vi "Arm.vi"(8 "error in (no error)":errorcluster, 11 "Shutter in":refnum<class "Shutter.lvclass">) -> (0 "error out":errorcluster, 2 "State":T1, 3 "Shutter out":refnum<class "Shutter.lvclass">)   [LabVIEW 2016, in "Shutter.lvclass"]
uses:
  Shutter.lvclass
  Controls/Shutter States.ctl
  Shutter.lvclass/Shutter.ctl
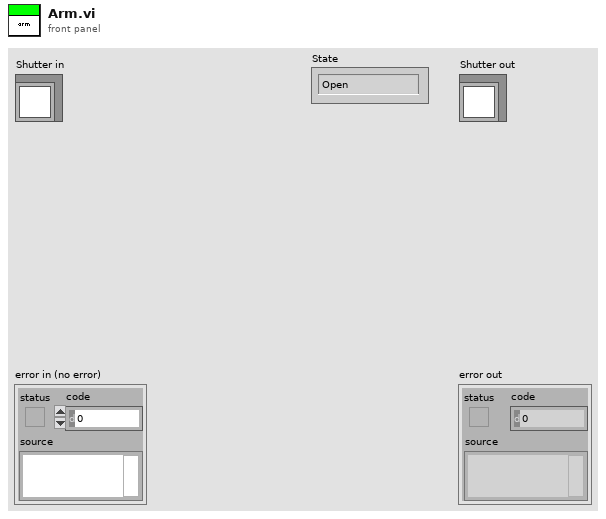
[diagram p1: front panel]
types:
  T1 = typedef "Shutter States.ctl" = enum16{"Open", "Close", "Wait", "Off", "Arm", "Idle"}
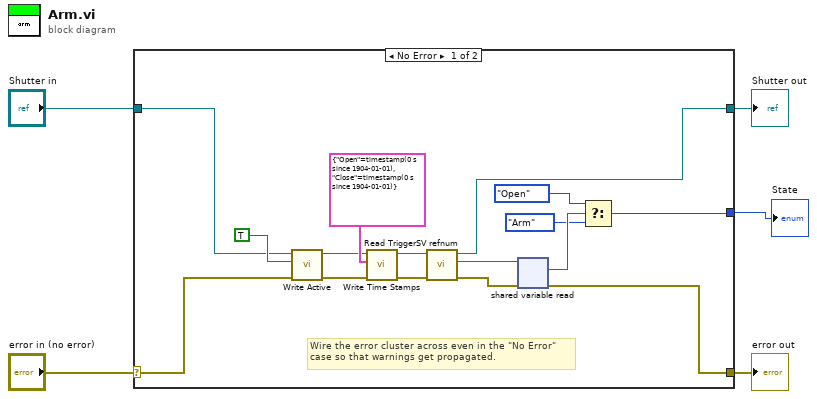
[diagram p0: block diagram]
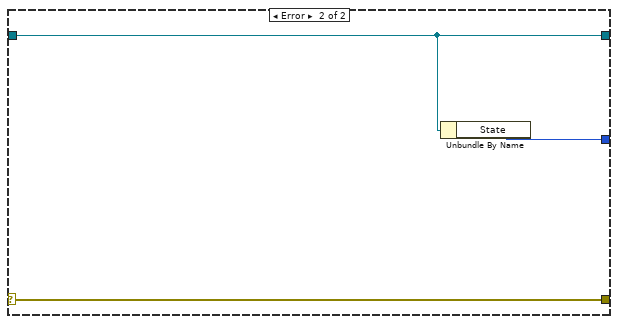
[diagram p2: hidden frame]
diagram:
  n1 = case shown="No Error" "error in (no error)" {
    selector: "error in (no error)" -> [w8 w24]
    tunnel: [w7 w24] -> w4
    tunnel: [w9 w22] -> w2
    tunnel: "Shutter in" -> [w10 w22]
    tunnel: [w6 w23] -> w1
    frame No Error {
      # "Wire the error cluster across even in the \"No Error\"\ncase so that warnings get propagated."
      n2 = call-dynamic "Write Active.vi"("error in (no error)"=w8, "Active"=TRUE, "Integrator in"=w10) -> ("error out"=w11:errorcluster, "Integrator out"=w12:refnum<class "Shutter.lvclass">)  [unwired: 7 in]
      n3 = call-dynamic "Write Time Stamps.vi"("error in (no error)"=w11, "Time Stamps"=cluster{"Open":timestamp, "Close":timestamp} {"Open"=timestamp(0 s since 1904-01-01), "Close"=timestamp(0 s since 1904-01-01)}, "Shutter in"=w12) -> ("error out"=w14:errorcluster, "Shutter out"=w15:refnum<class "Shutter.lvclass">)  [unwired: 7 in]
      n4 = call-dynamic "Read TriggerSV refnum.vi"("error in (no error)"=w14, "Shutter in"=w15) -> ("error out"=w17:errorcluster, "TriggerSV refnum"=w18:refnum<k21>, "Shutter out"=w9:refnum<class "Shutter.lvclass">)  [unwired: 7 in]
      n5 = shared-variable-read(w18, w17) -> (w7:errorcluster, w21:bool)  [unwired: 2 out]
      n6 = Select(t=Shutter_States."Open" ("State"), s=w21, f=Shutter_States."Arm") -> (s? t:f=w6:T1)
    }
    frame Error {
      n7 = Unbundle By Name(w22) -> ("State"=w23:T1)
    }
  }
  "error out" <- w4
  "Shutter out" <- w2
  "State" <- w1
